vi "Read Is on ConPane_.vi"(8 "error in (no error)":errorcluster, 11 "Control in":refnum<class "Control.lvclass">) -> (0 "error out":errorcluster, 2 "Is on ConPane?":bool, 3 "Control out":refnum<class "Control.lvclass">)   [LabVIEW 2020, in "VI Properties Editor.lvlib" / "Control.lvclass"]
doc: "Gets or sets whether the control is on the connector pane."
uses:
  Control.lvclass
  Control.lvclass/Control.ctl
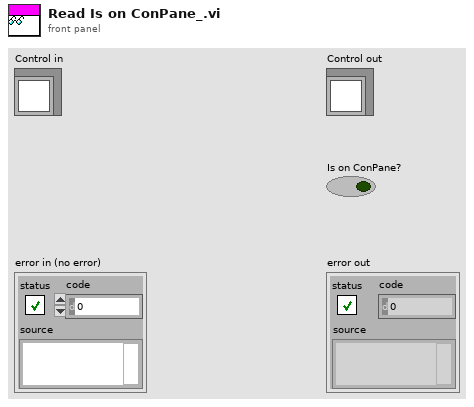
[diagram p1: front panel]
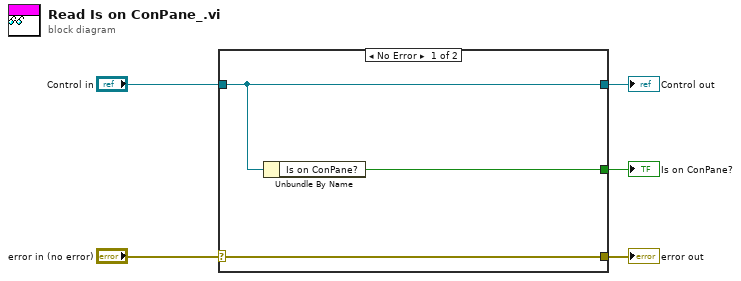
[diagram p0: block diagram]
diagram:
  n1 = case shown="No Error" "error in (no error)" {
    selector: "error in (no error)" -> [w8 w9]
    tunnel: [w8 w9] -> w4
    tunnel: [w7 w10] -> w2
    tunnel: "Control in" -> [w7 w10]
    tunnel: [w6 _] -> w1
    frame No Error {
      n2 = Unbundle By Name(w7) -> ("Is on ConPane?"=w6:bool)
    }
    frame Error {
    }
  }
  "error out" <- w4
  "Control out" <- w2
  "Is on ConPane?" <- w1
